vi "TestStand_Wait For Temperature Stability.vi"(7 "Timeout":dbl=120.0 caption="Time Target (s)" format="%#_g Seconds", 10 "Tolerance":dbl=0.1 format="%#_g °C", 11 "Temperature Target":dbl=37.5 caption="Target" format="%#_g °C") -> (0 "Error Out":errorcluster, 1 "Delta RTD_Target (°C)":dbl format="%#_g °C", 2 "RTD Temperature (°C)":dbl format="%#_g °C")   [LabVIEW 2010]
panel:
  in  "stop":bool
  out "Timeout?":string
  out "Temperature and Delta History":T1(graph)
  out "Temperature Target (°C)":dbl min=25.0 max=80.0 step=0.1 format="%#_g °C"
  out "Air Temperature (°C)":dbl min=25.0 max=80.0 step=0.1 format="%#_g °C"
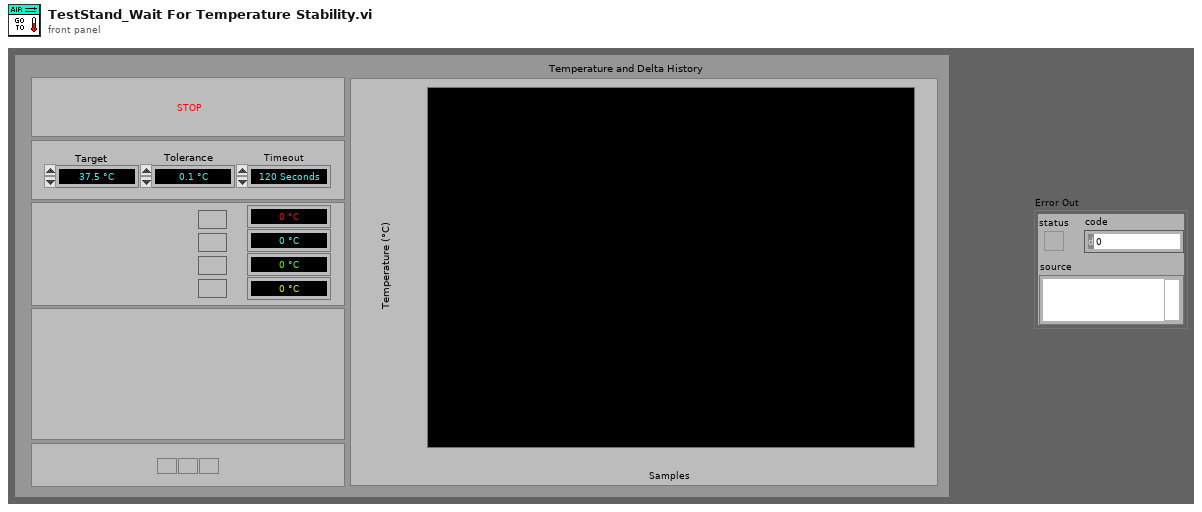
[diagram p1: front panel]
types:
  T1 = cluster{"Temperature Target":dbl, "Air Temperature (°C)":dbl, "Temperature (DegC)":dbl, dbl}
  T2 = cluster{"Temperature Target":dbl, "Air Temperature (°C)":dbl, "Temperature (DegC)":dbl, dbl}[]
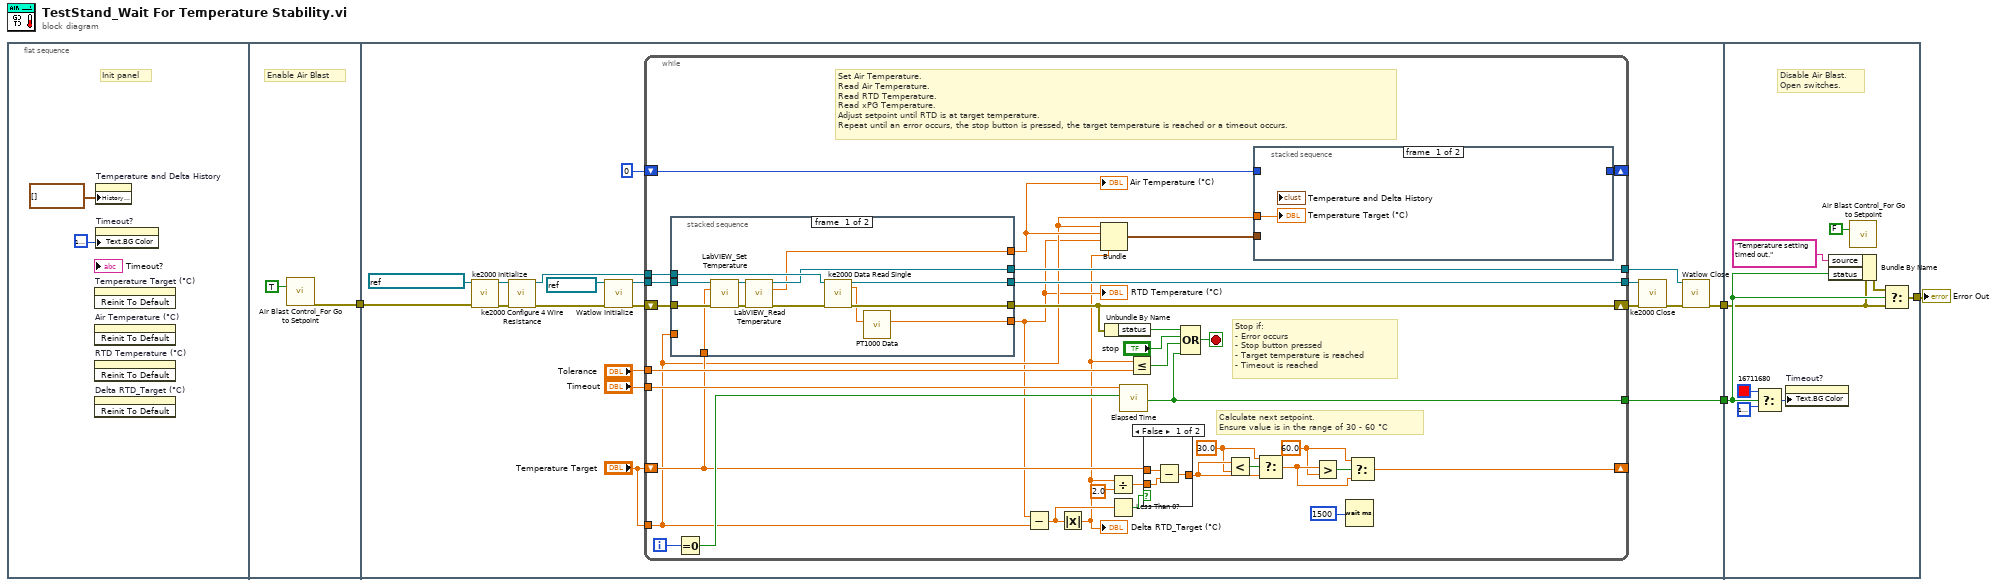
[diagram p0: block diagram]
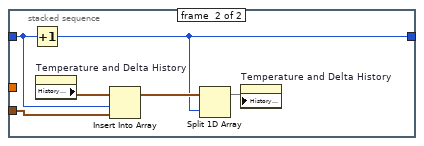
[diagram p2: hidden frame]
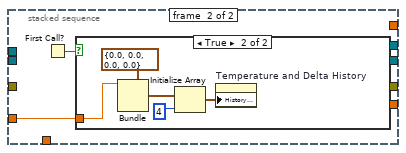
[diagram p3: hidden frame]
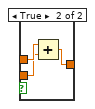
[diagram p5: hidden frame]
diagram:
  n1 = flat-sequence {
    tunnel: [w7] -> w3
    tunnel: [w19] -> w4
    tunnel: w3 -> [w22]
    tunnel: [w9] -> w2
    tunnel: w4 -> [w99]
    tunnel: [w100] -> w1
    tunnel: w2 -> [w97]
    frame #0 {
      # "Init panel"
      n2 = invoke on="Temperature Target (°C)" class="DigNum (strict)" method="Reinit To Default"() -> ()  [unwired: 3 in, 3 out]
      n3 = invoke on="Air Temperature (°C)" class="DigNum (strict)" method="Reinit To Default"() -> ()  [unwired: 3 in, 3 out]
      n4 = invoke on="RTD Temperature (°C)" class="DigNum (strict)" method="Reinit To Default"() -> ()  [unwired: 3 in, 3 out]
      n5 = invoke on="Delta RTD_Target (°C)" class="DigNum (strict)" method="Reinit To Default"() -> ()  [unwired: 3 in, 3 out]
      n6 = property on="Temperature and Delta History" class="WFChart (strict)"("History Data"=T2 []) -> ()  [unwired: 2 in, 2 out]
      n7 = property on="Timeout?" class="Str"("Text.BG Color"=u32 16777216) -> ()  [unwired: 2 in, 2 out]
    }
    frame #1 {
      # "Enable Air Blast"
      n8 = call "Air Blast Control_For Go to Setpoint.vi"("Enable/Disable"=TRUE) -> ("error out"=w7:errorcluster)  [unwired: 14 in]
    }
    frame #2 {
      n9 = call "ke2000 Initialize.vi"("VISA resource name"=refnum<visa-resource-name> "GPIB0::8::INSTR", "error in (no error)"=w22) -> ("VISA resource name out"=w26:refnum<visa-resource-name>, "error out"=w27:errorcluster)  [unwired: 16 in]
      n10 = call "ke2000 Configure 4 Wire Resistance.vi"("VISA resource name"=w26, "error in (no error)"=w27) -> ("VISA resource name out"=w25:refnum<visa-resource-name>, "error out"=w15:errorcluster)  [unwired: 16 in]
      n11 = call <instrlib>:"Watlow Initialize.vi"("Comms Port"=refnum<visa-resource-name> "COM7", "Error In"=w15) -> ("UUT Port 2"=w13:refnum<visa-resource-name>, "Error Out"=w14:errorcluster)  [unwired: 15 in, 1 out]
      n12 = while {
        tunnel: w25 -> [w54]
        tunnel: [w53] -> w24
        shift-right: [w43] -> _
        shift-left: "Temperature Target" -> [w40]
        tunnel: "Temperature Target" -> [w38]
        shift-right: [w57] -> w11
        shift-left: w14 -> [w58]
        tunnel: "Tolerance" -> [w59]
        tunnel: "Timeout" -> [w60]
        tunnel: [w31] -> w19
        shift-right: [w36] -> _
        shift-left: 0 -> [w37]
        tunnel: w13 -> [w35]
        tunnel: [w61] -> w12
        i -> [w30]
        stop <- w56 stop-if-true
        w42 = 60.0 ("y")
        w46 = 30.0 ("y")
        # "Stop if:\n- Error occurs\n- Stop button pressed\n- Target temperature is reached\n- Timeout is reached"
        # "Calculate next setpoint.\nEnsure value is in the range of 30 - 60 °C"
        # "Set Air Temperature.\nRead Air Temperature.\nRead RTD Temperature.\nRead xPG Temperature.\nAdjust setpoint until RTD is at target temperature.\nRepeat until an error occurs, the stop button is pressed, the target temperature is reached or a timeout occurs."
        n13 = stacked-sequence {
          tunnel: w58 -> [w82 _]
          tunnel: w40 -> [w81 _]
          tunnel: [w80 _] -> w57
          tunnel: [w71 _] -> w41
          tunnel: w54 -> [w79 _]
          tunnel: [w78 _] -> w53
          tunnel: [w77 _] -> w29
          tunnel: w38 -> [_ w84]
          tunnel: w35 -> [w73 _]
          tunnel: [w72 _] -> w61
          frame #0 {
            n14 = call "LabVIEW_Set Temperature.vi"("PC Comms Port"=w73, "Air Temperature Setpoint (°C)"=w81, "error in (no error)"=w82) -> ("PC Comms Port Out"=w74:refnum<visa-resource-name>, "error out"=w76:errorcluster)  [unwired: 11 in]
            n15 = call "LabVIEW_Read Temperature.vi"("PC Comms Port"=w74, "error in (no error)"=w76) -> ("PC Comms Port Out"=w72:refnum<visa-resource-name>, "Air Temperature (°C)"=w71:dbl, "error out"=w75:errorcluster)  [unwired: 11 in]
            n16 = call "ke2000 Data Read Single.vi"("VISA resource name"=w79, "error in (no error)"=w75) -> ("VISA resource name out"=w78:refnum<visa-resource-name>, "Measurement"=w70:dbl, "error out"=w80:errorcluster)  [unwired: 13 in, 2 out]
            n17 = call "PT1000 Data.vi"("Resistance (Ohms)"=w70) -> ("Temperature (DegC)"=w77:dbl)  [unwired: 10 in]
          }
          frame #1 {
            n18 = First Call?() -> (First Call?: T/F=w83:bool)
            n19 = case shown="True" w83 {
              tunnel: w84 -> [_ w87]
              frame False {
              }
              frame True {
                n20 = Bundle(cluster=T1 {"Temperature Target"=0.0, "Air Temperature (°C)"=0.0, "Temperature (DegC)"=0.0, 0.0} ("Temperature and Delta History"), "Temperature Target"=w87) -> (w89:T1)  [unwired: 3 in]
                n21 = Initialize Array(w89, 4 ("dimension size")) -> (w88:T2)
                n22 = property on="Temperature and Delta History" class="WFChart (strict)"("History Data"=w88) -> ()  [unwired: 2 in, 2 out]
              }
            }
          }
        }
        "RTD Temperature (°C)" <- w29
        "Air Temperature (°C)" <- w41
        n23 = Equal To 0?(x=w30) -> (x = 0?=w62:bool)
        n24 = Subtract(x=w29, y=w38) -> (x-y=w52:dbl)
        n25 = Absolute Value(x=w52) -> (abs(x)=w28:dbl)
        "Delta RTD_Target (°C)" <- w28
        n26 = Bundle("Temperature Target"=w38, "Air Temperature (°C)"=w41, "Temperature (DegC)"=w29, w28) -> (w39:T1)  [unwired: 1 in]
        n27 = Unbundle By Name(w57) -> ("status"=w34:bool)
        n28 = Divide(x=w28, y=2.0) -> (x/y=w49:dbl)
        n29 = Less Than 0?(x=w52) -> (x < 0?=w50:bool)
        n30 = call "Elapsed Time"("Time Target (s)"=w60, "Reset"=w62) -> ("Time has Elapsed"=w31:bool)  [unwired: 10 in, 7 out]
        n31 = Less Or Equal?(x=w28, y=w59) -> (x <= y?=w32:bool)
        n32 = case shown="False" w50 {
          tunnel: w40 -> [w91 w95]
          tunnel: [w92 w94] -> w47
          tunnel: w49 -> [w90 w93]
          frame False {
            n33 = Subtract(x=w91, y=w90) -> (x-y=w92:dbl)
          }
          frame True {
            n34 = Add(x=w95, y=w93) -> (x+y=w94:dbl)
          }
        }
        n35 = Compound Arithmetic op=OR(w34, "stop", w32, w31) -> (w56:bool)
        n36 = Less?(x=w47, y=w46) -> (x < y?=w48:bool)
        n37 = stacked-sequence {
          tunnel: w39 -> [_ w64]
          tunnel: w37 -> [_ w66]
          tunnel: w38 -> [w63 _]
          tunnel: [_ w65] -> w36
          frame #0 {
            "Temperature Target (°C)" <- w63
          }
          frame #1 {
            n38 = Increment(x=w66) -> (x+1=w65:i32)
            n39 = property on="Temperature and Delta History" class="WFChart (strict)"() -> ("History Data"=w69:T2)  [unwired: 2 in, 2 out]
            n40 = Insert Into Array(array=w69, index=w66, new element=w64) -> (w68:T2)
            n41 = Split 1D Array(array=w68, index=w65) -> (first subarray=w67:T2)  [unwired: 1 out]
            n42 = property on="Temperature and Delta History" class="WFChart (strict)"("History Data"=w67) -> ()  [unwired: 2 in, 2 out]
          }
        }
        n43 = Select(t=w46, s=w48, f=w47) -> (s? t:f=w44:dbl)
        n44 = Greater?(x=w44, y=w42) -> (0:w45:bool)
        n45 = Wait (ms)(milliseconds to wait=u32 1500) -> ()  [unwired: 1 out]
        n46 = Select(t=w42, s=w45, f=w44) -> (s? t:f=w43:dbl)
      }
      n47 = call "ke2000 Close.vi"("VISA resource name"=w24, "error in (no error)"=w11) -> ("error out"=w10:errorcluster)  [unwired: 17 in]
      n48 = call <instrlib>:"Watlow Close.vi"("PC Comms Port"=w12, "Error In"=w10) -> ("Error Out"=w9:errorcluster)  [unwired: 16 in, 1 out]
    }
    frame #3 {
      # "Disable Air Blast.\nOpen switches."
      n49 = Select(t=u32 16711680, s=w99, f=u32 16777216) -> (s? t:f=w102:u32)
      n50 = property on="Timeout?" class="Str"("Text.BG Color"=w102) -> ()  [unwired: 2 in, 2 out]
      n51 = Bundle By Name(cluster=w97, "source"="Temperature setting timed out.", "status"=w99) -> (w98:errorcluster)
      n52 = call "Air Blast Control_For Go to Setpoint.vi"("Enable/Disable"=FALSE) -> ()  [unwired: 14 in, 1 out]
      n53 = Select(t=w98, s=w99, f=w97) -> (s? t:f=w100:errorcluster)
    }
  }
  "Error Out" <- w1
